vi "server state machine.vi"(8 "results reporter":refnum<class "results reporter.lvclass">, 9 "execution system":T1=enum."standard", 10 "thread pool":refnum<class "thread pool.lvclass">, 11 "connection server in":refnum<class "connection server.lvclass">) -> ()   [LabVIEW 2015, in "connection server.lvclass"]
uses:
  connection server.lvclass
  taskpool/dispatcher/thread pool.lvclass
  taskpool/dispatcher/execution system.ctl
  taskpool/results reporter/results reporter.lvclass
  state.ctl
  communicator/communicator.lvclass/communicator.ctl
  message/communicator message.lvclass/communicator message.ctl
  connection server.lvclass/connection server.ctl
  communicator queue/identifying queue.lvclass/identifying queue.ctl
  communicator/communicator.lvclass
  communicator queue/identifying queue.lvclass
  message/set sender.vi
  message/communicator message.lvclass
  connection/connection maintainer.lvclass
  communicator manager/communicator manager.lvlib
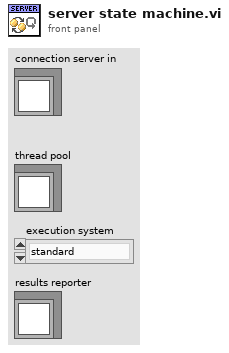
[diagram p1: front panel]
types:
  T1 = typedef "thread pool.lvclass/execution system.ctl" = enum32{"user interface", "standard", "instrument i/o", "data acquisition", "other 1", "other 2"}
  T2 = typedef "connection server.lvclass/state.ctl" = enum16{"start listening", "stop listening", "waiting"}
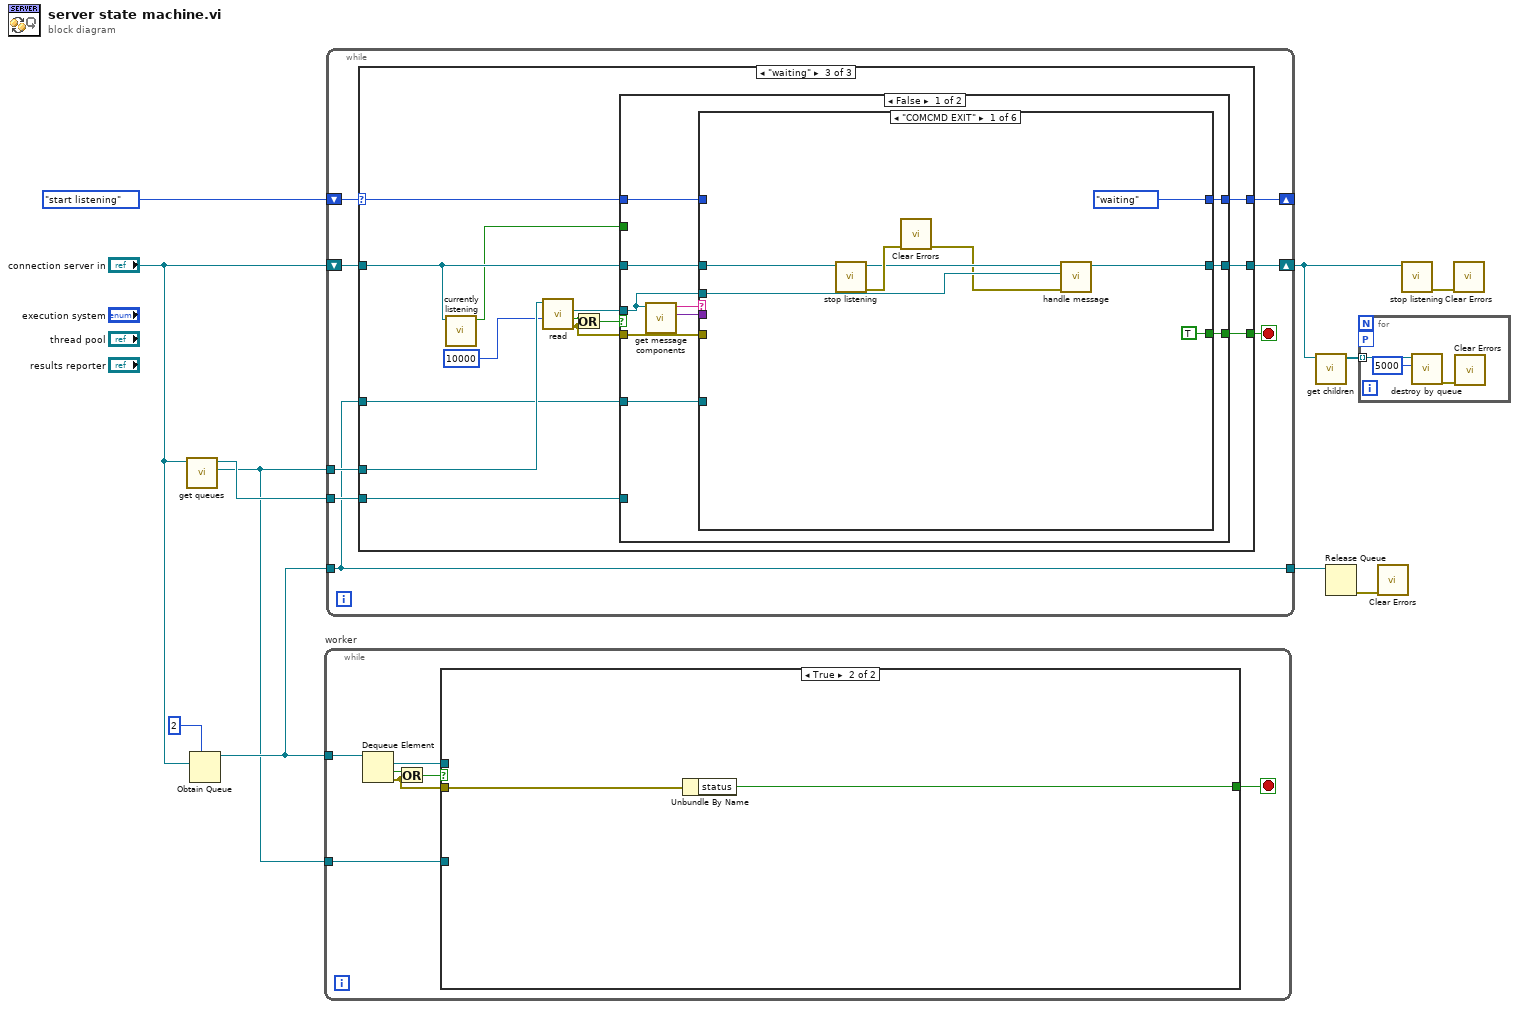
[diagram p0: block diagram]
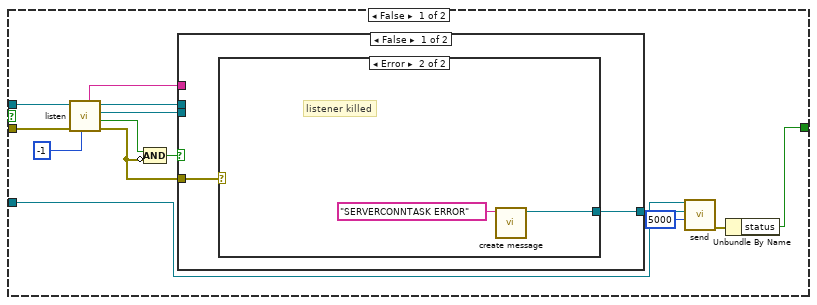
[diagram p2: hidden frame]
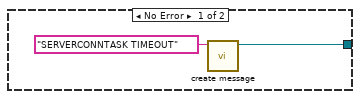
[diagram p3: hidden frame]
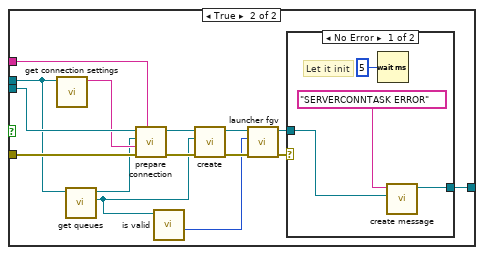
[diagram p4: hidden frame]
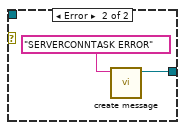
[diagram p5: hidden frame]
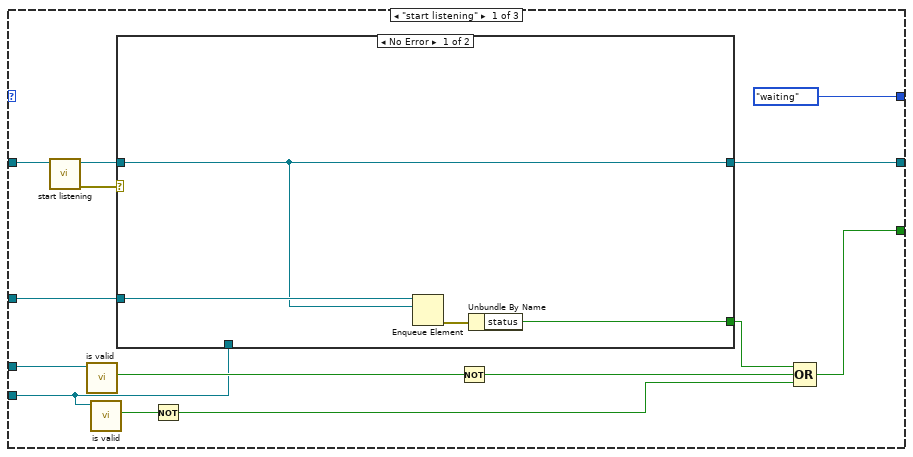
[diagram p6: hidden frame]
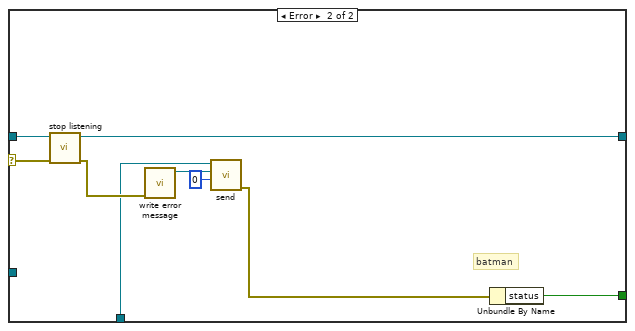
[diagram p7: hidden frame]
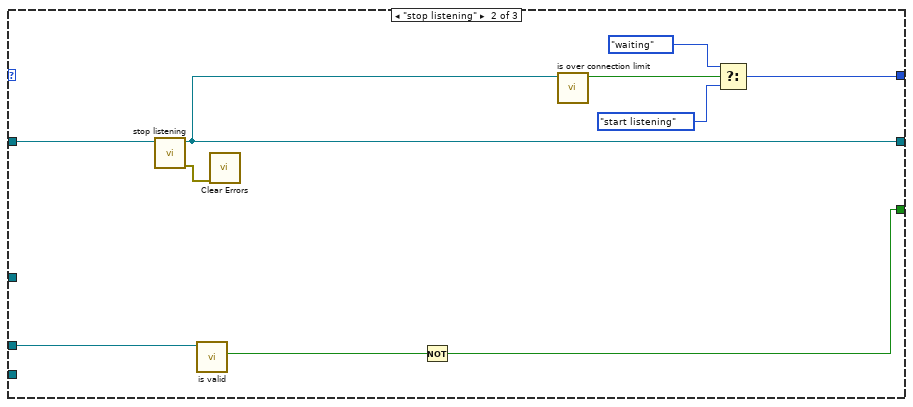
[diagram p8: hidden frame]
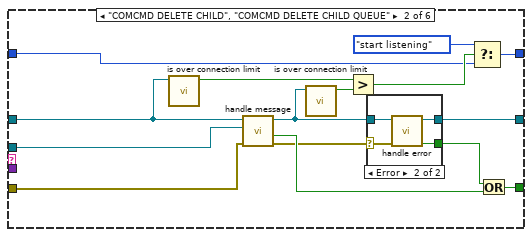
[diagram p9: hidden frame]
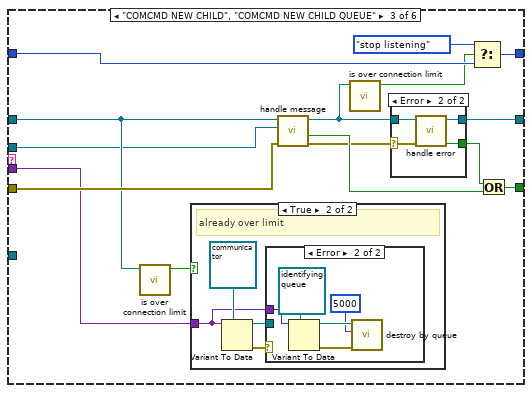
[diagram p11: hidden frame]
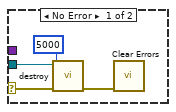
[diagram p13: hidden frame]
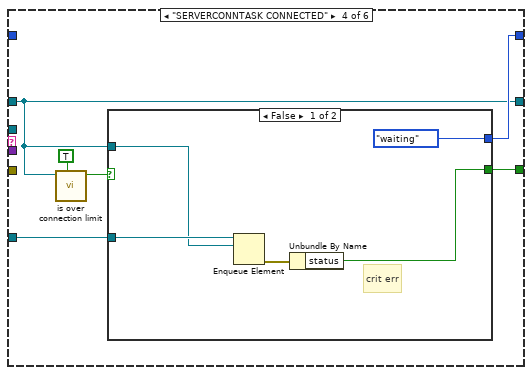
[diagram p15: hidden frame]
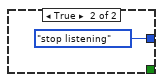
[diagram p16: hidden frame]
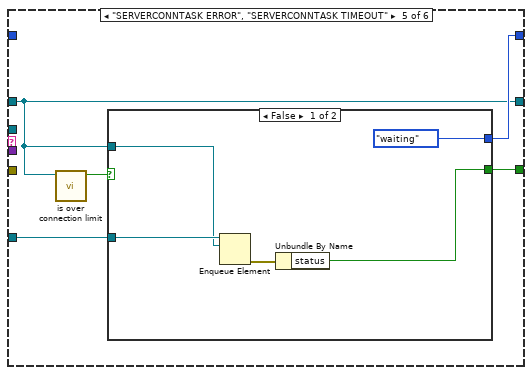
[diagram p17: hidden frame]
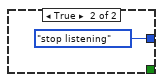
[diagram p18: hidden frame]
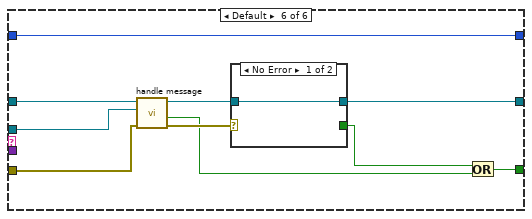
[diagram p19: hidden frame]
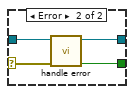
[diagram p20: hidden frame]
diagram:
  n1 = call "get queues.vi"("communicator in"="connection server in") -> ("to this"=w2:refnum<class "identifying queue.lvclass">, "to parent"=w10:refnum<class "identifying queue.lvclass">)  [unwired: 9 in]
  n2 = Obtain Queue(max queue size (-1, unlimited)=2, element data type="connection server in") -> (queue out=w5:refnum<queue>)  [unwired: 3 in, 2 out]
  n3 = while "worker" {
    tunnel: w5 -> [w18]
    tunnel: w2 -> [w12]
    stop <- w13 stop-if-true
    n4 = Dequeue Element(queue=w18) -> (element=w15:refnum<class "connection server.lvclass">, timed out?=w17:bool, error out=w14:errorcluster)  [unwired: 2 in, 1 out]
    n5 = Or(x=w17, y=w14) -> (x .or. y?=w16:bool)
    n6 = case shown="True" w16 {
      tunnel: w15 -> [w25 _]
      tunnel: w14 -> [w24 w61]
      tunnel: [w22 w60] -> w13
      tunnel: w12 -> [w21 _]
      frame False {
        n7 = call-dynamic "listen.vi"("timeout ms (10000)"=-1 ("timeout ms (wait forever: -1)"), "error in"=w24, "connection server in"=w25) -> ("error out"=w29:errorcluster, "valid?"=w27:bool, "new connection"=w30:refnum<class "connection maintainer.lvclass">, "connection server out"=w31:refnum<class "connection server.lvclass">, "client ID"=w32:string)  [unwired: 4 in]
        n8 = Compound Arithmetic op=AND(w27, invert w29) -> (w28:bool)
        n9 = case shown="False" w28 {
          tunnel: w29 -> [w33 w53]
          tunnel: w30 -> [_ w52]
          tunnel: w31 -> [_ w45]
          tunnel: w32 -> [_ w50]
          tunnel: [w34 w40] -> w20
          frame False {
            n10 = case shown="Error" w33 {
              tunnel: [w36 w37] -> w34
              frame No Error {
                n11 = call "create message.vi"("ID"="SERVERCONNTASK TIMEOUT") -> ("message"=w36:refnum<class "communicator message.lvclass">)  [unwired: 10 in]
              }
              frame Error {
                # "listener killed"
                n12 = call "create message.vi"("ID"="SERVERCONNTASK ERROR") -> ("message"=w37:refnum<class "communicator message.lvclass">)  [unwired: 10 in]
              }
            }
          }
          frame True {
            n13 = call "get connection settings.vi"("connection server in"=w45) -> ("connection string"=w51:string)  [unwired: 9 in, 1 out]
            n14 = call "get queues.vi"("communicator in"=w45) -> ("to this"=w43:refnum<class "identifying queue.lvclass">, "to parent"=w44:refnum<class "identifying queue.lvclass">)  [unwired: 9 in]
            n15 = call-dynamic "prepare connection.vi"("client string"=w50, "error in"=w53, "connection string"=w51, "queue manager"=w44, "connection in"=w52) -> ("error out"=w48:errorcluster, "connection out"=w49:refnum<class "connection maintainer.lvclass">)  [unwired: 5 in]
            n16 = call "is valid.vi"("identifying queue in"=w43) -> ("max queue size"=w42:i32)  [unwired: 9 in, 1 out]
            n17 = call "create.vi"("error in"=w48, "parent"=w43, "uninitialized communicator"=w49) -> ("error out"=w47:errorcluster, "communicator out"=w46:refnum<class "connection maintainer.lvclass">)  [unwired: 7 in]
            n18 = call "launcher fgv.vi"("error in"=w47, "queue size (1,10000)"=w42, "communicator in"=w46) -> ("error out"=w41:errorcluster, "initialized communicator"=w39:refnum<class "communicator.lvclass">)  [unwired: 7 in]
            n19 = case shown="No Error" w41 {
              tunnel: [w55 w58] -> w40
              tunnel: w39 -> [w54 _]
              frame No Error {
                # "Let it init"
                n20 = Wait (ms)(milliseconds to wait=u32 5) -> ()  [unwired: 1 out]
                n21 = call "create message.vi"("data"=w54, "ID"="SERVERCONNTASK ERROR") -> ("message"=w55:refnum<class "communicator message.lvclass">)  [unwired: 9 in]
              }
              frame Error {
                n22 = call "create message.vi"("ID"="SERVERCONNTASK ERROR") -> ("message"=w58:refnum<class "communicator message.lvclass">)  [unwired: 10 in]
              }
            }
          }
        }
        n23 = call "send.vi"("timeout in ms (-1)"=5000, "message"=w20, "message connection in"=w21) -> ("error out"=w23:errorcluster)  [unwired: 7 in, 1 out]
        n24 = Unbundle By Name(w23) -> ("status"=w22:bool)
      }
      frame True {
        n25 = Unbundle By Name(w61) -> ("status"=w60:bool)
      }
    }
  }
  n26 = while {
    shift-right: [w68] -> _
    shift-left: state."start listening" -> [w69]
    tunnel: w2 -> [w67]
    tunnel: w10 -> [w66]
    shift-right: [w64] -> w7
    shift-left: "connection server in" -> [w65]
    tunnel: w5 -> [w62]
    tunnel: [w62] -> w4
    stop <- w63 stop-if-true
    n27 = case shown="\"waiting\"" w69 {
      selector: w69 -> [_ _ w115]
      tunnel: [state."waiting" w97 w117] -> w68
      tunnel: w67 -> [w77 w104 w120]
      tunnel: w66 -> [w75 _ w109]
      tunnel: w65 -> [w83 w106 w113]
      tunnel: [w80 w101 w112] -> w64
      tunnel: [w74 w102 w110] -> w63
      tunnel: w62 -> [w70 _ w108]
      frame "start listening" {
        n28 = call-dynamic "start listening.vi"("connection server in"=w83) -> ("error out"=w82:errorcluster, "connection server out"=w81:refnum<class "connection server.lvclass">)  [unwired: 9 in]
        n29 = call "is valid.vi"("identifying queue in"=w77) -> ("valid?"=w79:bool)  [unwired: 9 in, 1 out]
        n30 = call "is valid.vi"("identifying queue in"=w75) -> ("valid?"=w76:bool)  [unwired: 9 in, 1 out]
        n31 = case shown="No Error" w82 {
          selector: w82 -> [_ w96]
          tunnel: w75 -> [_ w91]
          tunnel: w81 -> [w84 w95]
          tunnel: [w84 w94] -> w80
          tunnel: [w86 w89] -> w71
          tunnel: w70 -> [w85 _]
          frame No Error {
            n32 = Enqueue Element(queue=w85, element=w84) -> (error out=w87:errorcluster)  [unwired: 2 in, 2 out]
            n33 = Unbundle By Name(w87) -> ("status"=w86:bool)
          }
          frame Error {
            # "batman"
            n34 = call-dynamic "stop listening.vi"("error in"=w96, "connection server in"=w95) -> ("error out"=w93:errorcluster, "connection server out"=w94:refnum<class "connection server.lvclass">)  [unwired: 8 in]
            n35 = call "write error message.vi"("error in"=w93) -> ("element"=w92:refnum<class "communicator message.lvclass">)  [unwired: 10 in]
            n36 = call "send.vi"("timeout in ms (-1)"=0, "message"=w92, "message connection in"=w91) -> ("error out"=w88:errorcluster)  [unwired: 7 in, 1 out]
            n37 = Unbundle By Name(w88) -> ("status"=w89:bool)
          }
        }
        n38 = Not(x=w76) -> (.not. x?=w73:bool)
        n39 = Not(x=w79) -> (.not. x?=w78:bool)
        n40 = Compound Arithmetic op=OR(w71, w78, w73) -> (w74:bool)
      }
      frame "stop listening" {
        n41 = call-dynamic "stop listening.vi"("connection server in"=w106) -> ("error out"=w105:errorcluster, "connection server out"=w101:refnum<class "connection server.lvclass">)  [unwired: 9 in]
        n42 = call "is valid.vi"("identifying queue in"=w104) -> ("valid?"=w103:bool)  [unwired: 9 in, 1 out]
        n43 = call <vilib>:"Clear Errors.vi"("error in (no error)"=w105) -> ()  [unwired: 5 in, 2 out]
        n44 = Not(x=w103) -> (.not. x?=w102:bool)
        n45 = call "is over connection limit.vi"("connection server in"=w101) -> ("over limit?"=w100:bool)  [unwired: 10 in]
        n46 = Select(t=state."waiting", s=w100, f=state."start listening") -> (s? t:f=w97:T2)
      }
      frame "waiting" {
        n47 = call-dynamic "currently listening.vi"("connection server in"=w113) -> ("listening?"=w111:bool)  [unwired: 10 in]
        n48 = call "read.vi"("timeout in ms (-1)"=10000, "identifying queue in"=w120) -> ("error out"=w114:errorcluster, "timed out?"=w119:bool, "message"=w118:refnum<class "communicator message.lvclass">)  [unwired: 7 in]
        n49 = Or(x=w119, y=w114) -> (x .or. y?=w116:bool)
        n50 = case shown="False" w116 {
          tunnel: w118 -> [w124 _]
          tunnel: [w128 w230] -> w117
          tunnel: w115 -> [w127 _]
          tunnel: w114 -> [w130 w242]
          tunnel: [w129 w236] -> w110
          tunnel: w113 -> [w125 w240]
          tunnel: [w126 w240] -> w112
          tunnel: w111 -> [_ w232]
          tunnel: w109 -> [_ w234]
          tunnel: w108 -> [w121 _]
          frame False {
            n51 = call "get message components.vi"("message"=w124) -> ("data"=w122:variant, "ID"=w123:string)  [unwired: 9 in]
            n52 = case shown="\"COMCMD EXIT\"" w123 {
              tunnel: w130 -> [_ w149 w170 _ _ w218]
              tunnel: [TRUE ("status") w141 w164 w193 w205 w217] -> w129
              tunnel: [state."waiting" w153 w173 w195 w207 w224] -> w128
              tunnel: w127 -> [_ w150 w171 _ _ w224]
              tunnel: w122 -> [_ _ w159 _ _ _]
              tunnel: w124 -> [w132 w143 w166 _ _ w219]
              tunnel: [w133 w142 w165 w194 w206 w220] -> w126
              tunnel: w125 -> [w135 w147 w168 w194 w206 w221]
              tunnel: w121 -> [_ _ _ w192 w204 _]
              frame "COMCMD EXIT" {
                n53 = call-dynamic "stop listening.vi"("connection server in"=w135) -> ("error out"=w136:errorcluster, "connection server out"=w134:refnum<class "connection server.lvclass">)  [unwired: 9 in]
                n54 = call <vilib>:"Clear Errors.vi"("error in (no error)"=w136) -> ("error out"=w131:errorcluster)  [unwired: 5 in, 1 out]
                n55 = call-dynamic "handle message.vi"("error in"=w131, "message"=w132, "communicator in"=w134) -> ("communicator out"=w133:refnum<class "connection server.lvclass">)  [unwired: 6 in, 2 out]
              }
              frame "COMCMD DELETE CHILD", "COMCMD DELETE CHILD QUEUE" {
                n56 = call "is over connection limit.vi"("connection server in"=w147) -> ("over limit?"=w146:bool)  [unwired: 10 in]
                n57 = call-dynamic "handle message.vi"("error in"=w149, "message"=w143, "communicator in"=w147) -> ("error out"=w139:errorcluster, "stop"=w148:bool, "communicator out"=w145:refnum<class "connection server.lvclass">)  [unwired: 6 in]
                n58 = call "is over connection limit.vi"("connection server in"=w145) -> ("over limit?"=w144:bool)  [unwired: 10 in]
                n59 = Greater?(x=w146, y=w144) -> (0:w152:bool)
                n60 = case shown="Error" w139 {
                  selector: w139 -> [_ w155]
                  tunnel: w145 -> [w154 w158]
                  tunnel: [w154 w157] -> w142
                  tunnel: [_ w156] -> w140
                  frame No Error {
                  }
                  frame Error {
                    n61 = call-dynamic "handle error.vi"("error in"=w155, "communicator in"=w158) -> ("unrecoverable?"=w156:bool, "communicator out"=w157:refnum<class "connection server.lvclass">)  [unwired: 8 in]
                  }
                }
                n62 = Select(t=state."start listening", s=w152, f=w150) -> (s? t:f=w153:T2)
                n63 = Or(x=w140, y=w148) -> (x .or. y?=w141:bool)
              }
              frame "COMCMD NEW CHILD", "COMCMD NEW CHILD QUEUE" {
                n64 = call "is over connection limit.vi"("connection server in"=w168) -> ("over limit?"=w160:bool)  [unwired: 10 in]
                n65 = case shown="True" w160 {
                  tunnel: w159 -> [_ w174]
                  frame False {
                  }
                  frame True {
                    # "already over limit"
                    n66 = Variant To Data(type=refnum<class "communicator.lvclass"> refnum ("child"), Variant=w174) -> (data=w175:refnum<class "communicator.lvclass">, error out=w176:errorcluster)  [unwired: 1 in]
                    n67 = case shown="Error" w176 {
                      selector: w176 -> [w180 _]
                      tunnel: w175 -> [w181 _]
                      tunnel: w174 -> [_ w186]
                      frame No Error {
                        n68 = call-dynamic "destroy.vi"("error in"=w180, "timeout in ms (-1)"=5000, "communicator in"=w181) -> ("error out"=w178:errorcluster)  [unwired: 8 in]
                        n69 = call <vilib>:"Clear Errors.vi"("error in (no error)"=w178) -> ()  [unwired: 5 in, 2 out]
                      }
                      frame Error {
                        n70 = Variant To Data(type=refnum<class "identifying queue.lvclass"> refnum ("child"), Variant=w186) -> (data=w184:refnum<class "identifying queue.lvclass">, error out=w183:errorcluster)  [unwired: 1 in]
                        n71 = call "destroy by queue.vi"("error in"=w183, "timeout in ms (-1)"=5000, "queue"=w184) -> ()  [unwired: 7 in, 2 out]
                      }
                    }
                  }
                }
                n72 = call-dynamic "handle message.vi"("error in"=w170, "message"=w166, "communicator in"=w168) -> ("error out"=w162:errorcluster, "stop"=w169:bool, "communicator out"=w167:refnum<class "connection server.lvclass">)  [unwired: 6 in]
                n73 = call "is over connection limit.vi"("connection server in"=w167) -> ("over limit?"=w161:bool)  [unwired: 10 in]
                n74 = case shown="Error" w162 {
                  selector: w162 -> [_ w188]
                  tunnel: w167 -> [w187 w191]
                  tunnel: [w187 w190] -> w165
                  tunnel: [_ w189] -> w163
                  frame No Error {
                  }
                  frame Error {
                    n75 = call-dynamic "handle error.vi"("error in"=w188, "communicator in"=w191) -> ("unrecoverable?"=w189:bool, "communicator out"=w190:refnum<class "connection server.lvclass">)  [unwired: 8 in]
                  }
                }
                n76 = Select(t=state."stop listening", s=w161, f=w171) -> (s? t:f=w173:T2)
                n77 = Or(x=w163, y=w169) -> (x .or. y?=w164:bool)
              }
              frame "SERVERCONNTASK CONNECTED" {
                n78 = call "is over connection limit.vi"("precheck?"=TRUE, "connection server in"=w194) -> ("over limit?"=w196:bool)  [unwired: 9 in]
                n79 = case shown="False" w196 {
                  tunnel: [state."waiting" state."stop listening"] -> w195
                  tunnel: w194 -> [w198 _]
                  tunnel: [w202 _] -> w193
                  tunnel: w192 -> [w200 _]
                  frame False {
                    # "crit err"
                    n80 = Enqueue Element(queue=w200, element=w198) -> (error out=w199:errorcluster)  [unwired: 2 in, 2 out]
                    n81 = Unbundle By Name(w199) -> ("status"=w202:bool)
                  }
                  frame True {
                  }
                }
              }
              frame "SERVERCONNTASK ERROR", "SERVERCONNTASK TIMEOUT" {
                n82 = call "is over connection limit.vi"("connection server in"=w206) -> ("over limit?"=w208:bool)  [unwired: 10 in]
                n83 = case shown="False" w208 {
                  tunnel: [state."waiting" state."stop listening"] -> w207
                  tunnel: w206 -> [w209 _]
                  tunnel: [w211 _] -> w205
                  tunnel: w204 -> [w210 _]
                  frame False {
                    n84 = Enqueue Element(queue=w210, element=w209) -> (error out=w212:errorcluster)  [unwired: 2 in, 2 out]
                    n85 = Unbundle By Name(w212) -> ("status"=w211:bool)
                  }
                  frame True {
                  }
                }
              }
              frame Default {
                n86 = call-dynamic "handle message.vi"("error in"=w218, "message"=w219, "communicator in"=w221) -> ("error out"=w223:errorcluster, "stop"=w215:bool, "communicator out"=w222:refnum<class "connection server.lvclass">)  [unwired: 6 in]
                n87 = case shown="No Error" w223 {
                  selector: w223 -> [_ w227]
                  tunnel: [w225 w228] -> w220
                  tunnel: w222 -> [w225 w229]
                  tunnel: [_ w226] -> w216
                  frame No Error {
                  }
                  frame Error {
                    n88 = call-dynamic "handle error.vi"("error in"=w227, "communicator in"=w229) -> ("unrecoverable?"=w226:bool, "communicator out"=w228:refnum<class "connection server.lvclass">)  [unwired: 8 in]
                  }
                }
                n89 = Or(x=w216, y=w215) -> (x .or. y?=w217:bool)
              }
            }
          }
          frame True {
            n90 = call "is valid.vi"("identifying queue in"=w234) -> ("valid?"=w237:bool)  [unwired: 9 in, 1 out]
            n91 = call "is over connection limit.vi"("connection server in"=w240) -> ("over limit?"=w233:bool)  [unwired: 10 in]
            n92 = Not(x=w237) -> (.not. x?=w235:bool)
            n93 = Compound Arithmetic op=AND(invert w232, invert w233) -> (w231:bool)
            n94 = Unbundle By Name(w242) -> ("status"=w241:bool)
            n95 = Select(t=state."start listening" ("f"), s=w231, f=state."waiting") -> (s? t:f=w230:T2)
            n96 = Or(x=w241, y=w235) -> (x .or. y?=w236:bool)
          }
        }
      }
    }
  }
  n97 = call "get children.vi"("communicator in"=w7) -> ("children"=w8:refnum<class "identifying queue.lvclass">[])  [unwired: 10 in]
  n98 = Release Queue(queue=w4) -> (error out=w3:errorcluster)  [unwired: 2 in, 2 out]
  n99 = for {
    tunnel: w8 -> [w243] mode=indexing
    workers-P: _ -> [_]
    n100 = call "destroy by queue.vi"("timeout in ms (-1)"=5000, "queue"=w243) -> ("error out"=w245:errorcluster)  [unwired: 8 in, 1 out]
    n101 = call <vilib>:"Clear Errors.vi"("error in (no error)"=w245) -> ()  [unwired: 5 in, 2 out]
  }
  n102 = call <vilib>:"Clear Errors.vi"("error in (no error)"=w3) -> ()  [unwired: 5 in, 2 out]
  n103 = call-dynamic "stop listening.vi"("connection server in"=w7) -> ("error out"=w9:errorcluster)  [unwired: 9 in, 1 out]
  n104 = call <vilib>:"Clear Errors.vi"("error in (no error)"=w9) -> ()  [unwired: 5 in, 2 out]
